vi "写入固件.vi"(8 "错误输入":errorcluster, 10 "保留原配置":bool=TRUE, 11 "MB session in":refnum<class "MB_Master.lvclass">) -> (0 "error out":errorcluster, 3 "MB session out":refnum<class "MB_Master.lvclass">)   [LabVIEW 2016]
uses:
  <vilib>/Plasmionique/MB Master/MB_Master/MB_Master.lvclass
  <vilib>/NI/Progress Bar/Controls/Update Bar Actions.ctl
  <vilib>/NI/Progress Bar/Controls/Progress Bar Properties.ctl
  <vilib>/Plasmionique/MB Master/MB_Master_Serial/MB_Master_Serial.lvclass
  D:/Program Files (x86)/National Instruments/LabVIEW 2016/vi.lib/Plasmionique/MB Master/MB_Master/MB_Master.lvclass
  <vilib>/regexp/Match Regular Expression.xnode
  <vilib>/Plasmionique/MB Master/MB Master.lvlib
  <vilib>/NI/Progress Bar/Progress Bar.lvlib
panel:
  in  "引用选择":enum16{"MB引用", "自建引用"}(ring)
  in  "VISA Resource":refnum<visa-resource-name>
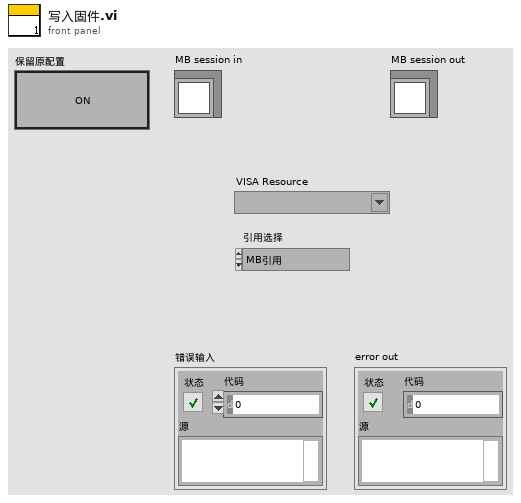
[diagram p1: front panel]
types:
  T1 = enum16{"open", "replace", "create", "open or create", "replace or create", "replace or create with confirmation"}
  T2 = enum16{"big-endian, network order", "native, host order", "little-endian"}
  T3 = typedef "Progress Bar.lvlib/Update Bar Actions.ctl" = enum16{"Add To Existing", "Set to Value"}
  T4 = cluster{"baud rate (bps)":u32, "stop bits":u16, "parity":u16, "flow control":u16, "timeout":u32, "retries":i32}
  T5 = typedef "Progress Bar.lvlib/Progress Bar Properties.ctl" = cluster{"Background Color":u32, "Installer Title":string, "Title Color":u32, "Action Text":string, "Text Color":u32, "Slider Value":u8, "Bar Color":u32, "Timeout":i32}
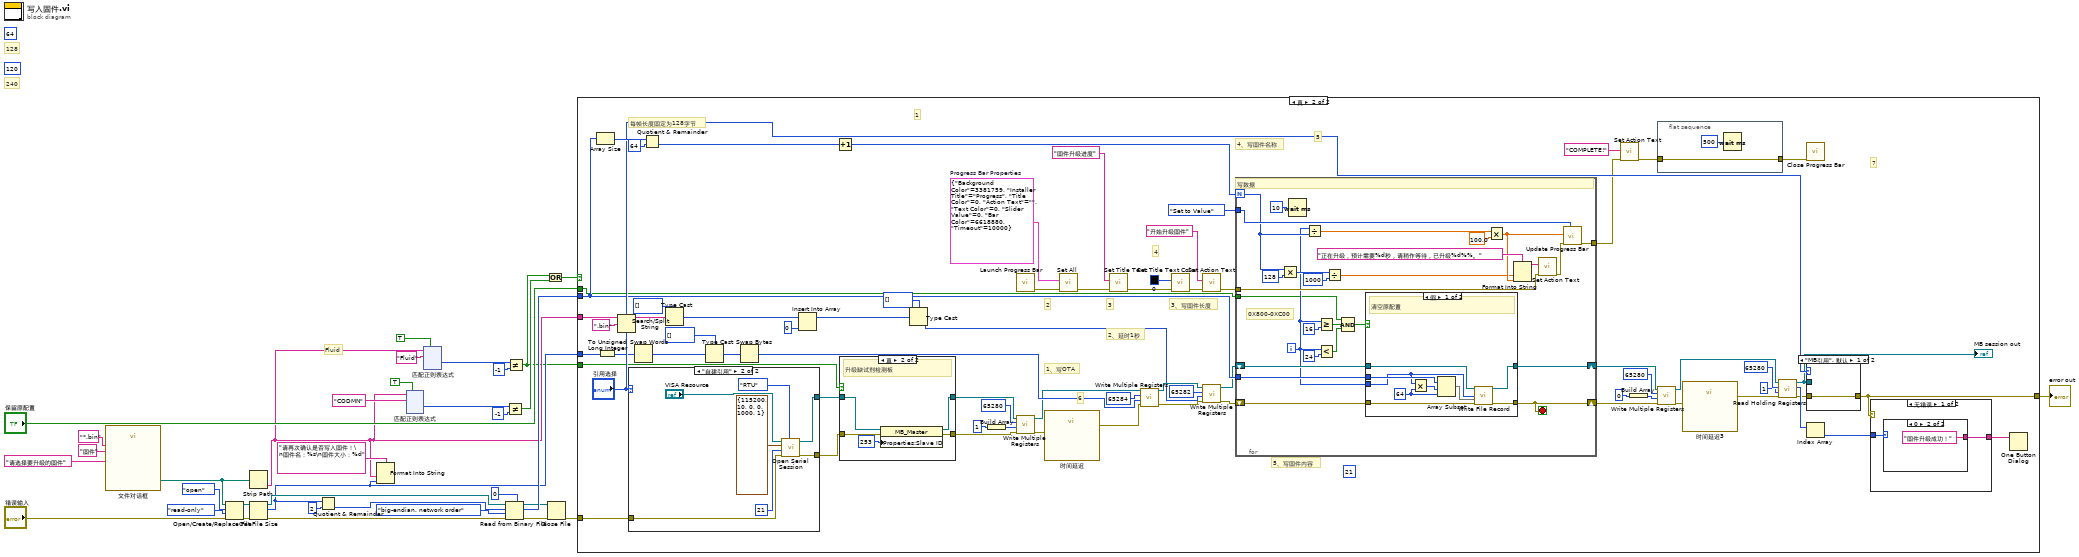
[diagram p0: block diagram]
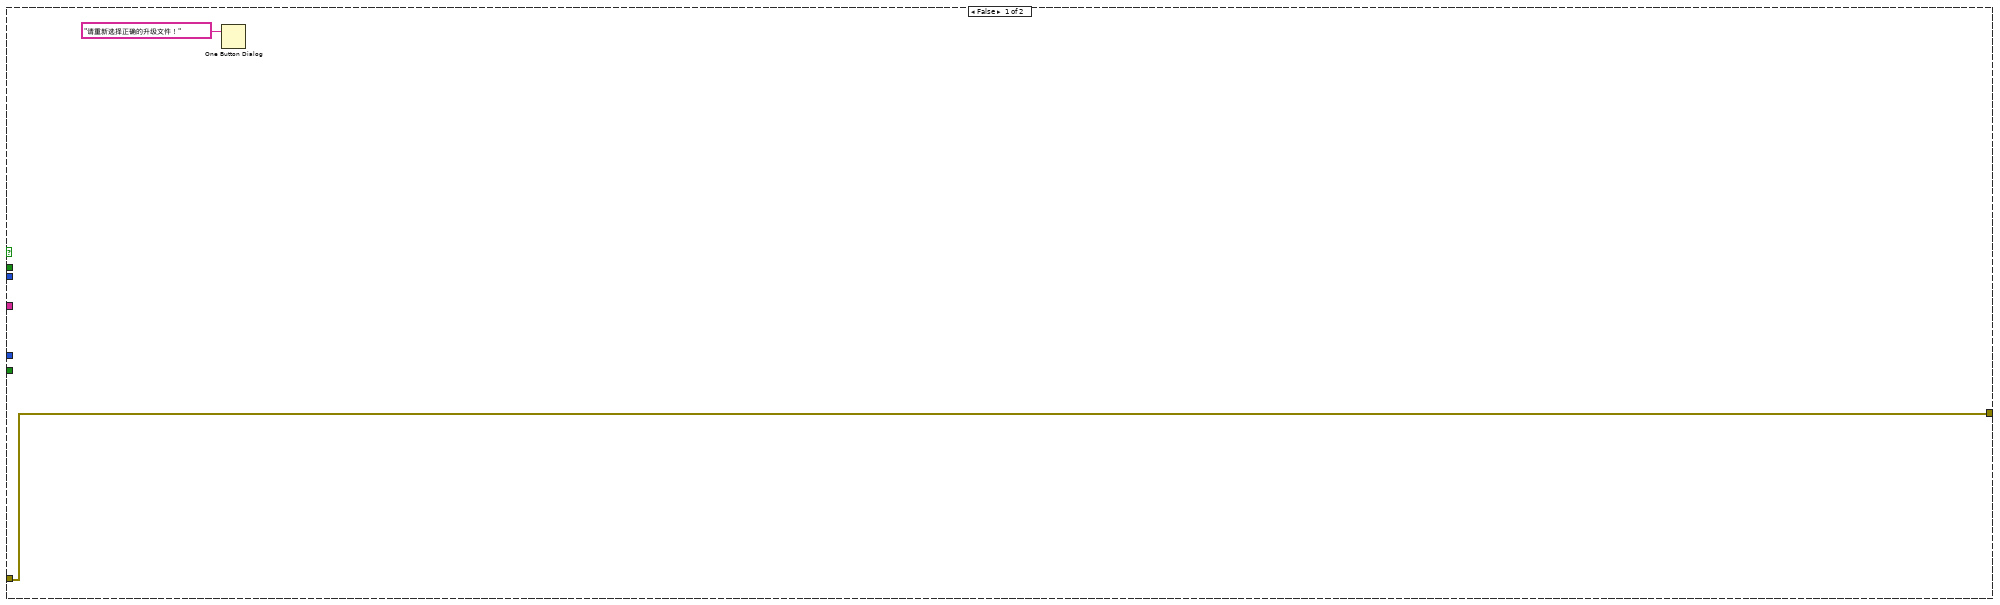
[diagram p2: hidden frame]
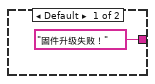
[diagram p4: hidden frame]
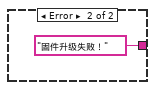
[diagram p5: hidden frame]
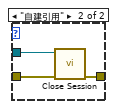
[diagram p6: hidden frame]
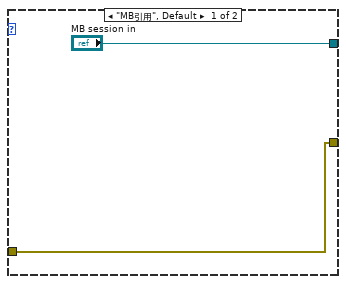
[diagram p7: hidden frame]
diagram:
  (unwired) 64 ("y")
  (unwired) 120 ("y")
  # "Fluid"
  # "240"
  # "128"
  n1 = call "文件对话框"("prompt"="请选择要升级的固件", "pattern (all files)"="*.bin", "pattern label"="固件") -> ("selected path"=w26:path)  [unwired: 9 in, 3 out]
  n2 = Open/Create/Replace File(file path (use dialog)=w26, error in="错误输入", operation (0:open)=T1."open" ("操作(0:open)"), access (0:read/write)=enum16{"read/write", "read-only", "write-only"}."read-only" ("权限(0:read/write)")) -> (refnum out=w25:refnum<file>, error out=w23:errorcluster)  [unwired: 2 in, 1 out]
  n3 = Strip Path(path=w26) -> (name=w3:string)  [unwired: 1 out]
  n4 = Get File Size(file=w25, error in=w23) -> (refnum out=w24:refnum<file>, size (in bytes)=w18:i64, 0:w22:errorcluster)
  n5 = Quotient & Remainder(x=w18, y=i64 2) -> (floor(x/y)=w20:i64)  [unwired: 1 out]
  n6 = Format Into String(format string="请再次确认是否写入固件！\n固件名：%s\n固件大小：%d" ("格式字符串"), w3, w18) -> ()  [unwired: 2 in, 2 out]
  n7 = xnode "匹配正则表达式"("输入字符串"=w3, "正则表达式"="CODMN", "忽略大小写？(F)"=TRUE) -> ("匹配后偏移量"=w13:i32)  [unwired: 3 in, 4 out]
  n8 = xnode "匹配正则表达式"("输入字符串"=w3, "正则表达式"="Fluid", "忽略大小写？(F)"=TRUE) -> ("匹配后偏移量"=w6:i32)  [unwired: 3 in, 4 out]
  n9 = Read from Binary File(5:u16 0, 8:w22, 9:T2."big-endian, network order" ("字节顺序(0:big-endian, network order)"), 10:w20, 11:w24) -> (0:w10:errorcluster, 2:w19:u16[], 3:w11:refnum<file>)  [unwired: 1 in, 1 out]
  n10 = Not Equal?(x=w13, y=-1) -> (x != y?=w8:bool)
  n11 = Not Equal?(x=w6, y=-1) -> (x != y?=w1:bool)
  n12 = Or(x=w1, y=w8) -> (x .or. y?=w2:bool)
  n13 = Close File(refnum=w11, error in=w10) -> (error out=w9:errorcluster)  [unwired: 1 out]
  n14 = case shown="真" w2 {
    tunnel: w19 -> [_ w78]
    tunnel: w3 -> [_ w91]
    tunnel: w9 -> [w37 w92]
    tunnel: [w37 w75] -> w29
    tunnel: w18 -> [_ w80]
    tunnel: "保留原配置" -> [_ w48]
    tunnel: w1 -> [_ w45]
    frame False {
      n15 = One Button Dialog(message="请重新选择正确的升级文件！" ("消息")) -> ()  [unwired: 1 in, 1 out]
    }
    frame True {
      w72 = T5 {"Background Color"=3381759, "Installer Title"="Progress", "Title Color"=0, "Action Text"="", "Text Color"=0, "Slider Value"=0, "Bar Color"=6618880, "Timeout"=10000}  # Progress Bar Properties
      (unwired) 21 ("Value")
      # "7"
      # "6"
      # "5"
      # "4"
      # "3"
      # "2"
      # "1"
      # "每帧长度固定为128字节"
      # "5、写固件内容"
      # "4、写固件名称"
      # "3、写固件长度"
      # "2、延时1秒"
      # "1、写OTA"
      n16 = Array Size(array=w78) -> (size(s)=w106:i32)
      n17 = To Unsigned Long Integer(number=w80) -> (unsigned 32bit integer=w77:u32)
      n18 = Search/Split String(string=w91, search string/char (-)=".bin" ("搜索字符串/字符(-)")) -> (substring before match=w89:string)  [unwired: 1 in, 2 out]
      n19 = case shown="\"自建引用\"" "引用选择" {
        tunnel: ["MB session in" w133] -> w47
        tunnel: w92 -> [w127 w132]
        tunnel: [w127 w131] -> w44
        frame "MB引用", Default {
        }
        frame "自建引用" {
          n20 = call <vilib>:"Open Serial Session.vi"("Mode (RTU)"=enum16{"RTU", "ASCII"}."RTU", "Error in"=w132, "Slave ID"=u8 21, "Serial Config"=T4 {"baud rate (bps)"=115200, "stop bits"=10, "parity"=0, "flow control"=0, "timeout"=1000, "retries"=1}, "VISA Resource"="VISA Resource") -> ("Error out"=w131:errorcluster, "MB_Serial session"=w133:refnum<class "MB_Master_Serial.lvclass">)  [unwired: 5 in]
        }
      }
      n21 = Swap Words(1:w77) -> (0:w76:u32)
      n22 = Quotient & Remainder(x=w106, y=64) -> (floor(x/y)=w107:i32)  [unwired: 1 out]
      n23 = Type Cast(type=u8[] [], x=w89) -> (*(type *) &x=w39:u8[])
      n24 = Type Cast(type=u16[] [], x=w76) -> (*(type *) &x=w100:u16[])
      n25 = Swap Bytes(anything=w100) -> (byte swapped=w99:u16[])
      n26 = Insert Into Array(array=w39, new element=u8 0 ("新元素/子数组")) -> (w40:u8[])  [unwired: 1 in]
      n27 = Increment(x=w107) -> (x+1=w79:i32)
      n28 = case shown="真" w45 {
        tunnel: w47 -> [w109 w114]
        tunnel: [w109 w113] -> w46
        tunnel: w44 -> [w108 w110]
        tunnel: [w108 w111] -> w43
        frame False {
          # "升级主板"
        }
        frame True {
          # "升级缺试剂检测板"
          n29 = property class="MB_Master"(reference=w114, error in=w110, "Properties:Slave ID"=u8 253 ("Slave ID")) -> (reference out=w113:refnum<class "MB_Master.lvclass">, error out=w111:errorcluster)
        }
      }
      n30 = Type Cast(type=u16[] [], x=w40) -> (*(type *) &x=w38:u16[])
      n31 = Build Array(u16 1 ("value")) -> (w93:u16[])
      n32 = call <vilib>:"Launch Progress Bar.vi"() -> ("error out"=w71:errorcluster)  [unwired: 10 in, 1 out]
      n33 = call <vilib>:"Write Multiple Registers.vi"("error in (no error)"=w43, "values"=w93, "starting address"=u16 65280, "MB session in"=w46) -> ("error out"=w102:errorcluster, "MB session out"=w83:refnum<class "MB_Master.lvclass">)  [unwired: 6 in]
      n34 = call "时间延迟"("error in (no error)"=w102) -> ("error out"=w84:errorcluster)  [unwired: 10 in]
      n35 = call <vilib>:"Set All.vi"("error in (no error)"=w71, "Progress Bar Properties (Default)"=w72) -> ("error out"=w65:errorcluster)  [unwired: 9 in]
      n36 = call <vilib>:"Set Title Text.vi"("error in (no error)"=w65, "Installer Title"="固件升级进度") -> ("error out"=w63:errorcluster)  [unwired: 9 in]
      n37 = call <vilib>:"Write Multiple Registers.vi"("error in (no error)"=w84, "values"=w99, "starting address"=u16 65284, "MB session in"=w83) -> ("error out"=w97:errorcluster, "MB session out"=w98:refnum<class "MB_Master.lvclass">)  [unwired: 6 in]
      n38 = call <vilib>:"Set Title Text Color.vi"("error in (no error)"=w63, "Color Box"=u32 0) -> ("error out"=w66:errorcluster)  [unwired: 9 in]
      n39 = call <vilib>:"Set Action Text.vi"("error in (no error)"=w66, "Action Text"="开始升级固件") -> ("error out"=w60:errorcluster)  [unwired: 9 in]
      n40 = call <vilib>:"Write Multiple Registers.vi"("error in (no error)"=w97, "values"=w38, "starting address"=u16 65282, "MB session in"=w98) -> ("error out"=w57:errorcluster, "MB session out"=w58:refnum<class "MB_Master.lvclass">)  [unwired: 6 in]
      n41 = for {
        N: w79 -> [w144]
        shift-right: [w159] -> w53
        shift-left: w58 -> [w161]
        shift-right: [w135] -> w49
        shift-left: w57 -> [w160]
        tunnel: w78 -> [w157]
        tunnel: Update_Bar_Actions."Set to Value" ("Action") -> [w156]
        tunnel: w60 -> [w154]
        tunnel: [w155] -> w59
        tunnel: w48 -> [w136]
        i -> [w141]
        stop <- w135 stop-if-true
        # "0X800-0XC00"
        # "写数据"
        n42 = Multiply(x=w144, y=128) -> (x*y=w148:i32)
        n43 = Wait (ms)(milliseconds to wait=u32 10) -> ()  [unwired: 1 out]
        n44 = Divide(x=w141, y=w144) -> (x/y=w150:dbl)
        n45 = Greater Or Equal?(x=w141, y=16) -> (x >= y?=w139:bool)
        n46 = Less?(x=w141, y=24) -> (x < y?=w138:bool)
        n47 = Divide(x=w148, y=u32 1000) -> (x/y=w145:dbl)
        n48 = Compound Arithmetic op=AND ("复合运算")(w136, w139, w138) -> (w137:bool)
        n49 = case shown="假" w137 {
          tunnel: w161 -> [w170 w172]
          tunnel: w160 -> [w169 w171]
          tunnel: [w168 w172] -> w159
          tunnel: [w167 w171] -> w135
          tunnel: w157 -> [w166 _]
          tunnel: w141 -> [w162 _]
          frame False {
            w164 = 64 ("长度")
            # "清空原配置"
            n50 = Multiply(x=w162, y=w164) -> (x*y=w163:i32)
            n51 = Array Subset(array=w166, index=w163, length=w164) -> (w165:u16[])
            n52 = call "Write File Record.vi"("MB session in"=w170, "Record Number"=w162, "values"=w165, "error in (no error)"=w169) -> ("MB session out"=w168:refnum<class "MB_Master.lvclass">, "error out"=w167:errorcluster)  [unwired: 10 in]
          }
          frame True {
            # "保留原配置"
          }
        }
        n53 = Multiply(x=w150, y=100.0) -> (x*y=w146:dbl)
        n54 = Format Into String(format string="正在升级，预计需要%d秒，请稍作等待，已升级%d%%。" ("格式字符串"), w145, w146) -> (resulting string=w151:string)  [unwired: 2 in, 1 out]
        n55 = call <vilib>:"Set Action Text.vi"("error in (no error)"=w154, "Action Text"=w151) -> ("error out"=w153:errorcluster)  [unwired: 9 in]
        n56 = call <vilib>:"Update Progress Bar.vi"("Action"=w156, "error in (no error)"=w153, "Value"=w146) -> ("error out"=w155:errorcluster)  [unwired: 8 in]
      }
      n57 = call <vilib>:"Set Action Text.vi"("error in (no error)"=w59, "Action Text"="COMPLETE!") -> ("error out"=w68:errorcluster)  [unwired: 9 in]
      n58 = Build Array(0 ("value")) -> (w54:i32[])
      n59 = flat-sequence {
        tunnel: w68 -> [w115]
        tunnel: [w115] -> w70
        frame #0 {
          n60 = Wait (ms)(milliseconds to wait=u32 500) -> ()  [unwired: 1 out]
        }
      }
      n61 = call <vilib>:"Write Multiple Registers.vi"("error in (no error)"=w49, "values"=w54, "starting address"=u16 65280, "MB session in"=w53) -> ("error out"=w51:errorcluster, "MB session out"=w52:refnum<class "MB_Master.lvclass">)  [unwired: 6 in]
      n62 = call "时间延迟3"("error in (no error)"=w51) -> ("error out"=w50:errorcluster)  [unwired: 10 in]
      n63 = call <vilib>:"Read Holding Registers.vi"("error in (no error)"=w50, "quantity"=u16 1, "starting address"=u16 65280, "MB session in"=w52) -> ("error out"=w81:errorcluster, "Registers"=w85:u16[], "MB session out"=w82:refnum<class "MB_Master.lvclass">)  [unwired: 5 in]
      "MB session out" <- w82
      n64 = call <vilib>:"Close Progress Bar.vi"("error in (no error)"=w70) -> ()  [unwired: 9 in, 2 out]
      n65 = case shown="\"MB引用\", 默认" "引用选择" {
        tunnel: w82 -> [_ w125]
        tunnel: w81 -> [w122 w124]
        tunnel: [w122 w123] -> w75
        frame "MB引用", Default {
        }
        frame "自建引用" {
          n66 = call-dynamic "Close Session.vi"("error in (no error)"=w124, "MB session in"=w125) -> ("error out"=w123:errorcluster)  [unwired: 9 in]
        }
      }
      n67 = Index Array(array=w85) -> (element=w74:u16)  [unwired: 1 in]
      n68 = case shown="无错误" w75 {
        tunnel: w74 -> [w118 _]
        tunnel: [w117 "固件升级失败！"] -> w73
        frame No Error {
          n69 = case shown="0" w118 {
            tunnel: ["固件升级失败！" "固件升级成功！"] -> w117
            frame Default {
            }
            frame 0 {
            }
          }
        }
        frame Error {
        }
      }
      n70 = One Button Dialog(message=w73) -> ()  [unwired: 1 in, 1 out]
    }
  }
  "error out" <- w29
